vi "Poly_WriteDigitalOut.vi"   [LabVIEW 2012]
doc: "Writes the value of \"Variable In\" to the specified digital \"Channel\"."
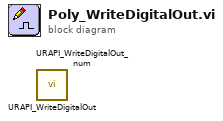
[diagram p0: block diagram]
diagram:
  n1 = call <userlib>:"URAPI_WriteDigitalOut.vi"() -> ()  [unwired: 4 in, 2 out]
  n2 = call <userlib>:"URAPI_WriteDigitalOut_num.vi"() -> ()  [unwired: 4 in, 2 out]
